vi "Master Setup Update Status.vi"(4 "Function":T1(ring), 6 "Progress Bar Refnum":refnum<vi>, 7 "Master Setup List Refnum":refnum<vi>) -> ()   [LabVIEW 2017]
panel:
  in  "Max Wait Time (ms)":u32=90000
  out "File Opened":bool[](array[boolean])
  out "Titles":string[](array[string])
  out "Files to Open":bool[](array[boolean])
  out "Elapsed Time (ms)":u32
  out "Update Loop Rate":u32
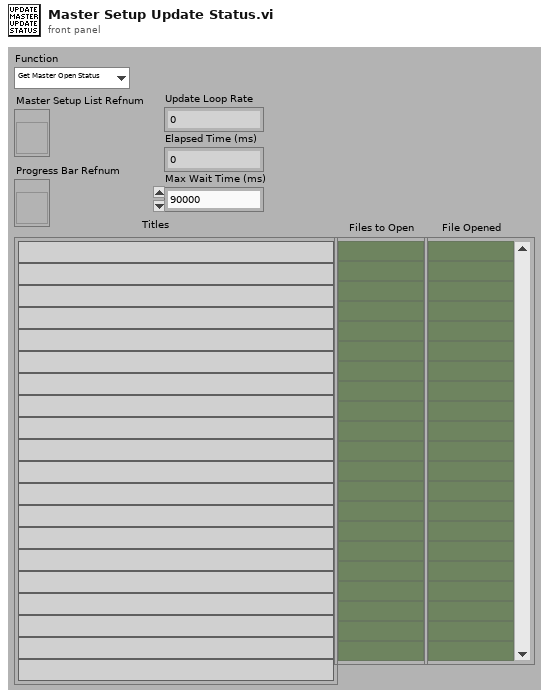
[diagram p1: front panel]
types:
  T1 = enum16{"Get Master Open Status", "Get Master Save Status"}
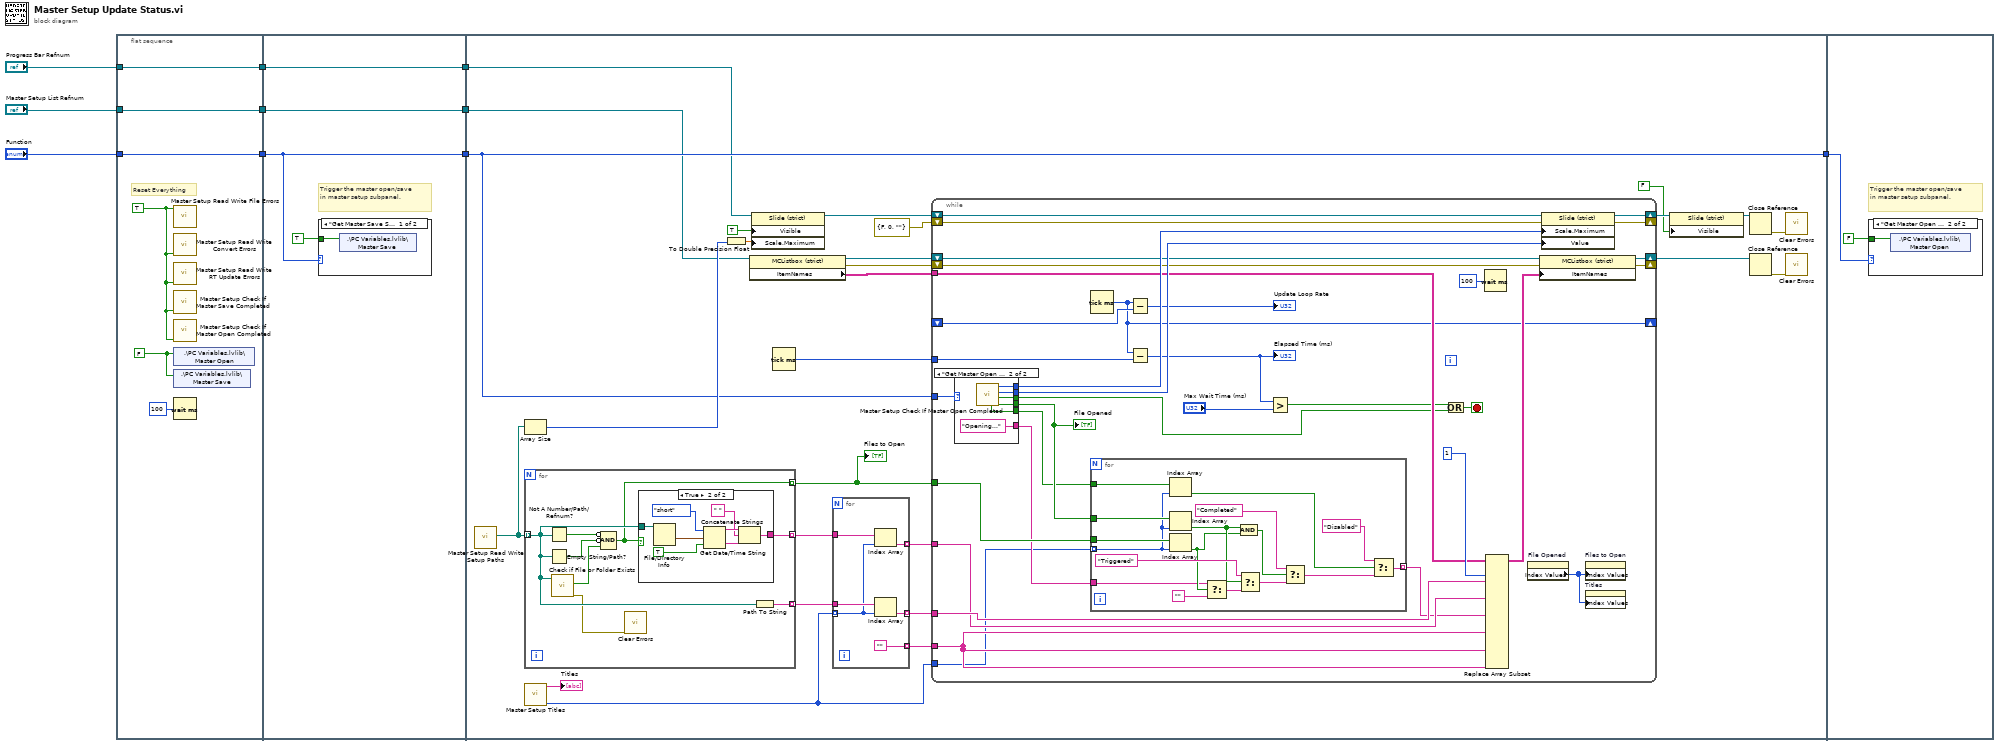
[diagram p0: block diagram]
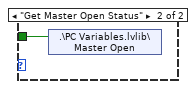
[diagram p2: hidden frame]
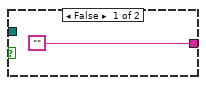
[diagram p3: hidden frame]
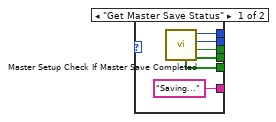
[diagram p4: hidden frame]
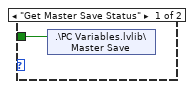
[diagram p5: hidden frame]
diagram:
  n1 = flat-sequence {
    tunnel: [w13] -> w10
    tunnel: "Function" -> [w13]
    tunnel: [w12] -> w5
    tunnel: "Progress Bar Refnum" -> [w12]
    tunnel: [w11] -> w2
    tunnel: "Master Setup List Refnum" -> [w11]
    tunnel: w10 -> [w19]
    tunnel: [w19] -> w8
    tunnel: [w18] -> w6
    tunnel: w5 -> [w18]
    tunnel: [w17] -> w3
    tunnel: w2 -> [w17]
    tunnel: w8 -> [w26]
    tunnel: [w26] -> w7
    tunnel: w6 -> [w25]
    tunnel: w3 -> [w24]
    tunnel: w7 -> [w136]
    frame #0 {
      w15 = FALSE ("Master Open")
      w16 = TRUE ("Reset")
      # "Reset Everything"
      n2 = call "Master Setup Read Write File Errors.vi"("Reset"=w16) -> ()  [unwired: 9 in, 2 out]
      n3 = call "Master Setup Read Write Convert Errors.vi"("Reset"=w16) -> ()  [unwired: 9 in, 2 out]
      n4 = call "Master Setup Read Write RT Update Errors.vi"("Reset"=w16) -> ()  [unwired: 8 in, 3 out]
      n5 = call "Master Setup Check If Master Save Completed.vi"("Reset"=w16) -> ()  [unwired: 6 in, 5 out]
      n6 = call "Master Setup Check If Master Open Completed.vi"("Reset"=w16) -> ()  [unwired: 6 in, 5 out]
      n7 = shared-variable ".\\PC Variables.lvlib\\Master Open"(w15) -> ()  [unwired: 1 in, 1 out]
      n8 = shared-variable ".\\PC Variables.lvlib\\Master Save"(w15) -> ()  [unwired: 1 in, 1 out]
      n9 = Wait (ms)(milliseconds to wait=u32 100) -> ()  [unwired: 1 out]
    }
    frame #1 {
      # "Trigger the master open/save in master setup subpanel."
      n10 = case shown="\"Get Master Save Status\"" w19 {
        tunnel: TRUE ("Master Save") -> [w21 w22]
        frame "Get Master Save Status" {
          n11 = shared-variable ".\\PC Variables.lvlib\\Master Save"(w21) -> ()  [unwired: 1 in, 1 out]
        }
        frame "Get Master Open Status" {
          n12 = shared-variable ".\\PC Variables.lvlib\\Master Open"(w22) -> ()  [unwired: 1 in, 1 out]
        }
      }
    }
    frame #2 {
      n13 = call "Master Setup Read Write Setup Paths.vi"() -> ("New Setup Paths"=w34:path[])  [unwired: 7 in, 4 out]
      n14 = Array Size(array=w34) -> (size(s)=w33:i32)
      n15 = for {
        tunnel: w34 -> [w59] mode=indexing
        tunnel: [w56] -> w27 mode=indexing
        tunnel: [w63] -> w39 mode=indexing
        tunnel: [w57] -> w40 mode=indexing
        n16 = Not A Number/Path/Refnum?(number/path/refnum=w59) -> (NaN/Path/Refnum?=w60:bool)
        n17 = Empty String/Path?(string/path=w59) -> (empty?=w62:bool)
        n18 = call <vilib>:"Check if File or Folder Exists.vi"("path"=w59) -> ("error out"=w58:errorcluster, "file or folder exists?"=w61:bool)  [unwired: 8 in, 1 out]
        n19 = Compound Arithmetic op=AND(invert w60, invert w62, w61) -> (w56:bool)
        n20 = call <vilib>:"Clear Errors.vi"("error in (no error)"=w58) -> ()  [unwired: 5 in, 2 out]
        n21 = case shown="True" w56 {
          tunnel: ["" w72] -> w57
          tunnel: w59 -> [_ w71]
          frame False {
          }
          frame True {
            n22 = File/Directory Info(path=w71) -> (last mod=w70:timestamp)  [unwired: 1 in, 6 out]
            n23 = Get Date/Time String(date format (0)=enum16{"short", "long", "abbreviated"}."short", seconds (now)=w70, want seconds? (F)=TRUE) -> (date string=w68:string, time string=w67:string)
            n24 = Concatenate Strings(w68, " " ("string"), w67) -> (w72:string)
          }
        }
        n25 = Path To String(path=w59) -> (string=w63:string)
      }
      "Files to Open" <- w27
      n26 = call "Master Setup Titles.vi"() -> ("Sorted Titles Indices"=w23:i32[], "Setup Description w/Numbers"=→"Titles":string[])  [unwired: 6 in, 4 out]
      n27 = To Double Precision Float(number=w33) -> (double precision float=w32:dbl)
      n28 = property class="MCListbox (strict)"(reference=w24) -> (reference out=w45:refnum<vi>, error out=w41:errorcluster, "ItemNames"=w44:string[][])  [unwired: 1 in]
      n29 = property class="Slide (strict)"(reference=w25, "Visible"=TRUE, "Scale.Maximum"=w32) -> (reference out=w35:refnum<vi>)  [unwired: 1 in, 1 out]
      n30 = Tick Count (ms)() -> (millisecond timer value=w43:u32)
      n31 = for {
        tunnel: w40 -> [w55]
        tunnel: w23 -> [w52] mode=indexing
        tunnel: [w54] -> w37 mode=indexing
        tunnel: w39 -> [w53]
        tunnel: [w51] -> w38 mode=indexing
        tunnel: [""] -> w36 mode=indexing
        n32 = Index Array(array=w55, index=w52) -> (element=w54:string)
        n33 = Index Array(array=w53, index=w52) -> (element=w51:string)
      }
      n34 = while {
        shift-right: [w88] -> _
        shift-left: _ -> [w100]
        tunnel: w27 -> [w84]
        shift-right: [w98] -> w30
        shift-left: w35 -> [w99]
        shift-right: [w97] -> w49
        shift-left: w45 -> [w92]
        shift-right: [w96] -> _
        shift-left: errorcluster {"status"=FALSE, "code"=0, "source"=""} ("error out") -> [w95]
        shift-right: [w93] -> _
        shift-left: w41 -> [w94]
        tunnel: w44 -> [w91]
        tunnel: w43 -> [w87]
        tunnel: w23 -> [w73]
        tunnel: w38 -> [w83]
        tunnel: w37 -> [w82]
        tunnel: w36 -> [w80]
        tunnel: w26 -> [w77]
        stop <- w90 stop-if-true
        n35 = case shown="\"Get Master Open Status\", Default" w77 {
          tunnel: [w112 w118] -> w104
          tunnel: [w111 w117] -> w103
          tunnel: [w110 w116] -> w79
          tunnel: [w109 w115] -> w78
          tunnel: ["Saving..." ("f") "Opening..." ("f")] -> w76
          tunnel: [w107 w113] -> w75
          frame "Get Master Save Status" {
            n36 = call "Master Setup Check If Master Save Completed.vi"() -> ("Master Save Status"=w110:bool[], "Master All Saved"=w109:bool, "Current Files Saved"=w112:i32, "Files to Save"=w111:i32, "Master Save Disabled List"=w107:bool[])  [unwired: 7 in]
          }
          frame "Get Master Open Status", Default {
            n37 = call "Master Setup Check If Master Open Completed.vi"() -> ("Master Open Status"=w116:bool[], "Master All Opened"=w115:bool, "Current Files Opened"=w118:i32, "Files to Open"=w117:i32, "Master Open Disabled List"=w113:bool[])  [unwired: 7 in]
          }
        }
        "File Opened" <- w79
        n38 = Tick Count (ms)() -> (millisecond timer value=w88:u32)
        n39 = for {
          tunnel: w79 -> [w135]
          tunnel: w73 -> [w121] mode=indexing
          tunnel: w84 -> [w131]
          tunnel: [w122] -> w81 mode=indexing
          tunnel: w76 -> [w125]
          tunnel: w75 -> [w120]
          n40 = Index Array(array=w120, index=w121) -> (element=w119:bool)
          n41 = Index Array(array=w135, index=w121) -> (element=w129:bool)
          n42 = Index Array(array=w131, index=w121) -> (element=w128:bool)
          n43 = Select(t=w125, s=w128, f="") -> (s? t:f=w133:string)
          n44 = And(x=w129, y=w128) -> (x .and. y?=w127:bool)
          n45 = Select(t="Triggered" ("Setup Description"), s=w129, f=w133) -> (s? t:f=w130:string)
          n46 = Select(t="Completed", s=w127, f=w130) -> (s? t:f=w123:string)
          n47 = Select(t="Disabled", s=w119, f=w123) -> (s? t:f=w122:string)
        }
        n48 = Subtract(x=w88, y=w100) -> (x-y=→"Update Loop Rate":u32)
        n49 = Subtract(x=w88, y=w87) -> (x-y=w74:u32)
        "Elapsed Time (ms)" <- w74
        n50 = Greater?(x=w74, y="Max Wait Time (ms)") -> (0:w89:bool)
        n51 = Or(x=w89, y=w78) -> (x .or. y?=w90:bool)
        n52 = Wait (ms)(milliseconds to wait=u32 100) -> ()  [unwired: 1 out]
        n53 = Replace Array Subset(array=w91, new element #1=w83, index (col) #1=1 ("disabled index (col)"), new element #2=w82, new element #3=w81, new element #4=w80, new element #5=w80, new element #6=w80) -> (w105:string[][])  [unwired: 11 in]
        n54 = property on="File Opened" class="Arr (strict)"() -> ("Index Values"=w85:u32[])  [unwired: 2 in, 2 out]
        n55 = property on="Property Node" class="MCListbox (strict)"(reference=w92, error in=w94, "ItemNames"=w105) -> (reference out=w97:refnum<vi>, error out=w93:errorcluster)
        n56 = property on="Property Node" class="Slide (strict)"(reference=w99, error in=w95, "Scale.Maximum"=w103, "Value"=w104) -> (reference out=w98:refnum<vi>, error out=w96:errorcluster)
        n57 = property on="Files to Open" class="Arr (strict)"("Index Values"=w85) -> ()  [unwired: 2 in, 2 out]
        n58 = property on="Titles" class="Arr (strict)"("Index Values"=w85) -> ()  [unwired: 2 in, 2 out]
      }
      n59 = property class="Slide (strict)"(reference=w30, "Visible"=FALSE) -> (reference out=w29:refnum<vi>)  [unwired: 1 in, 1 out]
      n60 = Close Reference(reference=w29) -> (error out=w47:errorcluster)  [unwired: 1 in]
      n61 = Close Reference(reference=w49) -> (error out=w46:errorcluster)  [unwired: 1 in]
      n62 = call <vilib>:"Clear Errors.vi"("error in (no error)"=w47) -> ()  [unwired: 5 in, 2 out]
      n63 = call <vilib>:"Clear Errors.vi"("error in (no error)"=w46) -> ()  [unwired: 5 in, 2 out]
    }
    frame #3 {
      # "Trigger the master open/save in master setup subpanel."
      n64 = case shown="\"Get Master Open Status\"" w136 {
        tunnel: FALSE ("Master Save") -> [w138 w139]
        frame "Get Master Save Status" {
          n65 = shared-variable ".\\PC Variables.lvlib\\Master Save"(w138) -> ()  [unwired: 1 in, 1 out]
        }
        frame "Get Master Open Status" {
          n66 = shared-variable ".\\PC Variables.lvlib\\Master Open"(w139) -> ()  [unwired: 1 in, 1 out]
        }
      }
    }
  }
